vi "Flatten Value.vi"(8 "error in":errorcluster, 11 "2D Int In":refnum<class "2D Int.lvclass">) -> (0 "error out":errorcluster, 1 "Value":string, 3 "2D Int Out":refnum<class "2D Int.lvclass">)   [LabVIEW 2020, in "NI_VIAnCFGDataStructure.lvlib" / "2D Int.lvclass"]
doc: "Dynamic dispatch interface for flattening Tree Data classes to string."
uses:
  <vilib>/addons/analyzer/VIAnCFGDataStructure/Data Types/2D Int/2D Int.lvclass
  <vilib>/addons/analyzer/VIAnCFGDataStructure/Data Types/2D Int/2D Int.lvclass/2D Int.ctl
  <vilib>/addons/analyzer/VIAnCFGDataStructure/Tree Manager/Tree.lvclass
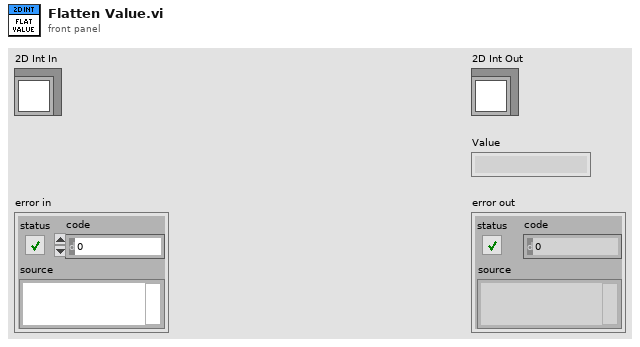
[diagram p1: front panel]
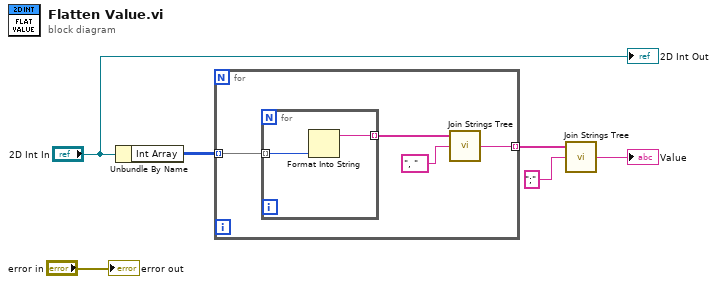
[diagram p0: block diagram]
diagram:
  n1 = Unbundle By Name("2D Int In") -> ("Int Array"=w3:i64[][])
  n2 = for {
    tunnel: w3 -> [w10] mode=indexing
    tunnel: [w8] -> w4 mode=indexing
    n3 = for {
      tunnel: w10 -> [w12] mode=indexing
      tunnel: [w11] -> w9 mode=indexing
      n4 = Format Into String(w12) -> (resulting string=w11:string)  [unwired: 3 in, 1 out]
    }
    n5 = call <vilib>:"Join Strings Tree.vi"("Separator (,)"=", ", "Strings In"=w9) -> ("String"=w8:string)  [unwired: 1 in]
  }
  n6 = call <vilib>:"Join Strings Tree.vi"("Separator (,)"=";", "Strings In"=w4) -> ("String"=→"Value":string)  [unwired: 1 in]
  "2D Int Out" <- "2D Int In"
  "error out" <- "error in"
